vi "Get Center Wavelength.vi"(11 "Array":dbl[](array[numeric])) -> (2 "Numeric":dbl, 3 "center wavelength":dbl)   [LabVIEW 2019, in "Spectrometer Calibration.lvlib"]
uses:
  Spectrometer Calibration.lvlib
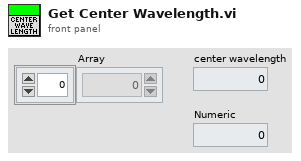
[diagram p1: front panel]
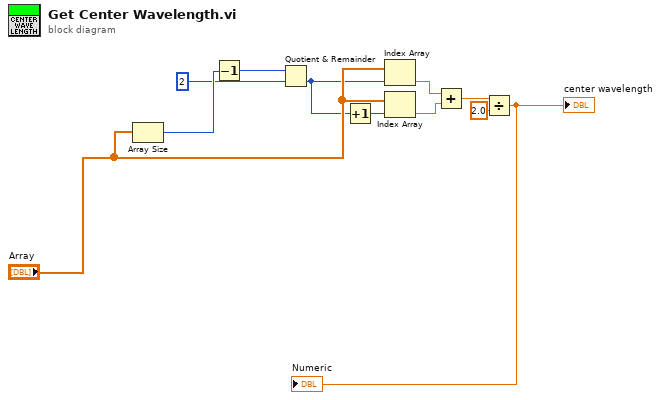
[diagram p0: block diagram]
diagram:
  n1 = Array Size(array="Array") -> (size(s)=w11:i32)
  n2 = Decrement(x=w11) -> (x-1=w2:i32)
  n3 = Quotient & Remainder(x=w2, y=2) -> (floor(x/y)=w3:i32)  [unwired: 1 out]
  n4 = Increment(x=w3) -> (x+1=w4:i32)
  n5 = Index Array(array="Array", index=w3) -> (element=w5:dbl)
  n6 = Index Array(array="Array", index=w4) -> (element=w6:dbl)
  n7 = Add(x=w5, y=w6) -> (x+y=w7:dbl)
  n8 = Divide(x=w7, y=2.0) -> (x/y=→"center wavelength" →"Numeric":dbl)
